vi "DVRLV2.vi"(0 "data value reference in":refnum<data-value>, 11 "error in":errorcluster, 13 "Operations":T1) -> (4 "data value reference out":refnum<data-value>, 15 "error out":errorcluster)   [LabVIEW 2023]
uses:
  Controls/LV2Operations.ctl
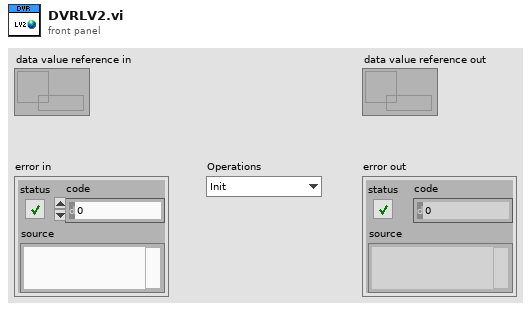
[diagram p1: front panel]
types:
  T1 = typedef "LV2Operations.ctl" = enum16{"Init", "Read", "Write"}
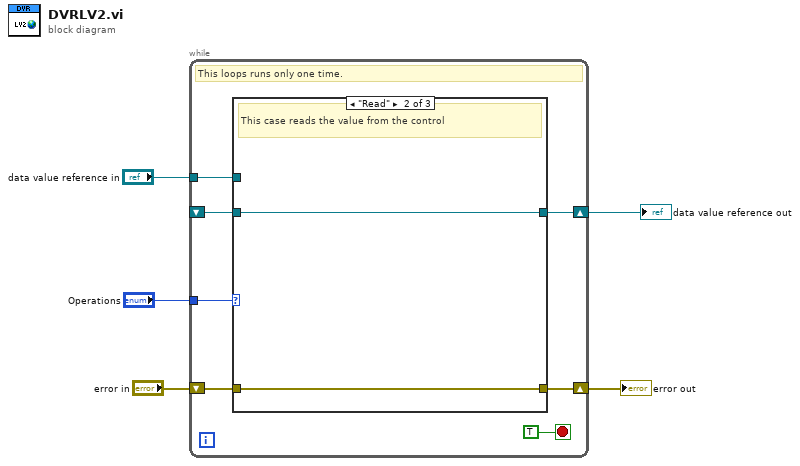
[diagram p0: block diagram]
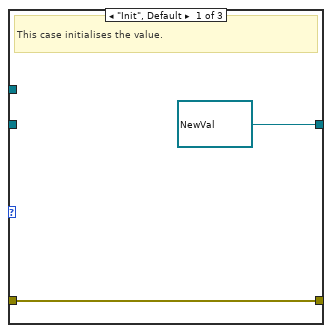
[diagram p2: hidden frame]
diagram:
  n1 = while {
    tunnel: "Operations" -> [w11]
    shift-right: [w9] -> w3
    shift-left: "error in" -> [w10]
    tunnel: "data value reference in" -> [w8]
    shift-right: [w6] -> w1
    shift-left: _ -> [w7]
    stop <- TRUE stop-if-true
    # "This loops runs only one time."
    n2 = case shown="\"Read\"" w11 {
      tunnel: w10 -> [w14 w16 w18]
      tunnel: [w14 w16 w18] -> w9
      tunnel: w8 -> [_ _ w17]
      tunnel: w7 -> [_ w15 _]
      tunnel: [refnum<data-value> refnum ("data value reference in") w15 w17] -> w6
      frame "Init", Default {
        # "This case initialises the value."
      }
      frame "Read" {
        # "This case reads the value from the control"
      }
      frame "Write" {
        # "This case writes value to the indicator"
      }
    }
  }
  "error out" <- w3
  "data value reference out" <- w1
